vi "Get Child Texts.vi"(10 "Item":string, 11 "Process Tree View Model in":refnum<class "Process Tree View Model.lvclass">) -> (3 "Texts":string[](array[string]))   [LabVIEW 2020, in "Process Tree View Model.lvclass"]
uses:
  Process Tree View Model.lvclass
  Process Tree View Model.lvclass/Process Tree View Model.ctl
  Debug Data/Debug Data.lvclass/Debug Data.ctl
  Debug Data/Debug Data.lvclass
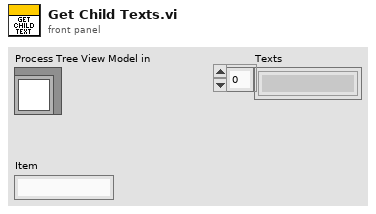
[diagram p1: front panel]
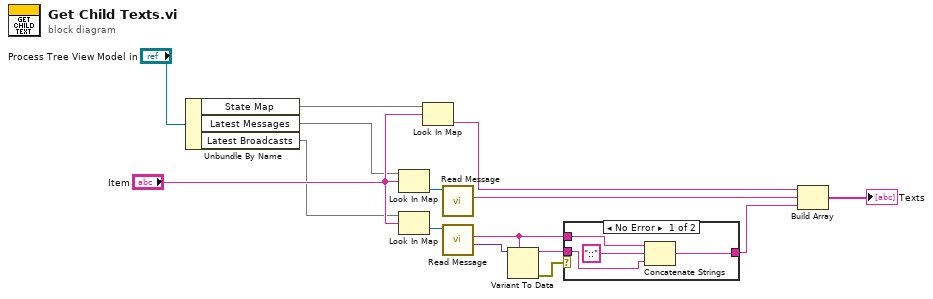
[diagram p0: block diagram]
diagram:
  n1 = Unbundle By Name("Process Tree View Model in") -> ("State Map"=w6:map{string, string}, "Latest Messages"=w9:map{string, refnum<class "Debug Data.lvclass">}, "Latest Broadcasts"=w13:map{string, refnum<class "Debug Data.lvclass">})
  n2 = Look In Map(map=w9, key="Item") -> (value=w10:refnum<class "Debug Data.lvclass">)  [unwired: 1 in, 1 out]
  n3 = Look In Map(map=w13, key="Item") -> (value=w14:refnum<class "Debug Data.lvclass">)  [unwired: 1 in, 1 out]
  n4 = Look In Map(map=w6, key="Item") -> (value=w7:string)  [unwired: 1 in, 1 out]
  n5 = call "Read Message.vi"("Debug Data in"=w10) -> ("Message"=w11:string)  [unwired: 8 in, 2 out]
  n6 = call "Read Message.vi"("Debug Data in"=w14) -> ("Message Data"=w3:variant, "Message"=w1:string)  [unwired: 8 in, 1 out]
  n7 = Variant To Data(type=w1, Variant=w3) -> (data=w4:string, error out=w5:errorcluster)  [unwired: 1 in]
  n8 = case shown="No Error" w5 {
    tunnel: w4 -> [w17 _]
    tunnel: w1 -> [w19 w20]
    tunnel: [w16 w20] -> w2
    frame No Error {
      n9 = Concatenate Strings(w19, "::" ("string"), w17) -> (w16:string)
    }
    frame Error {
    }
  }
  n10 = Build Array(w7, w11, w2) -> (→"Texts":string[])
